vi "GDSIconEditor_MaskIcon.vi"(6 "BgIcon":u8[][](array[numeric]), 8 "ColorsOkayforiconToBeOnTopOf":u8[](array[numeric]), 9 "BgIconOffset":cluster{"X":i32, "Y":i32}, 10 "BgIconMask":u8[](array[numeric]), 11 "IconIn":u8[][](array[numeric])) -> (3 "IconOut":u8[][](array[numeric]))   [LabVIEW 2014]
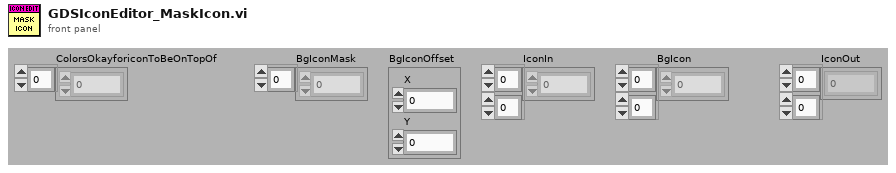
[diagram p1: front panel]
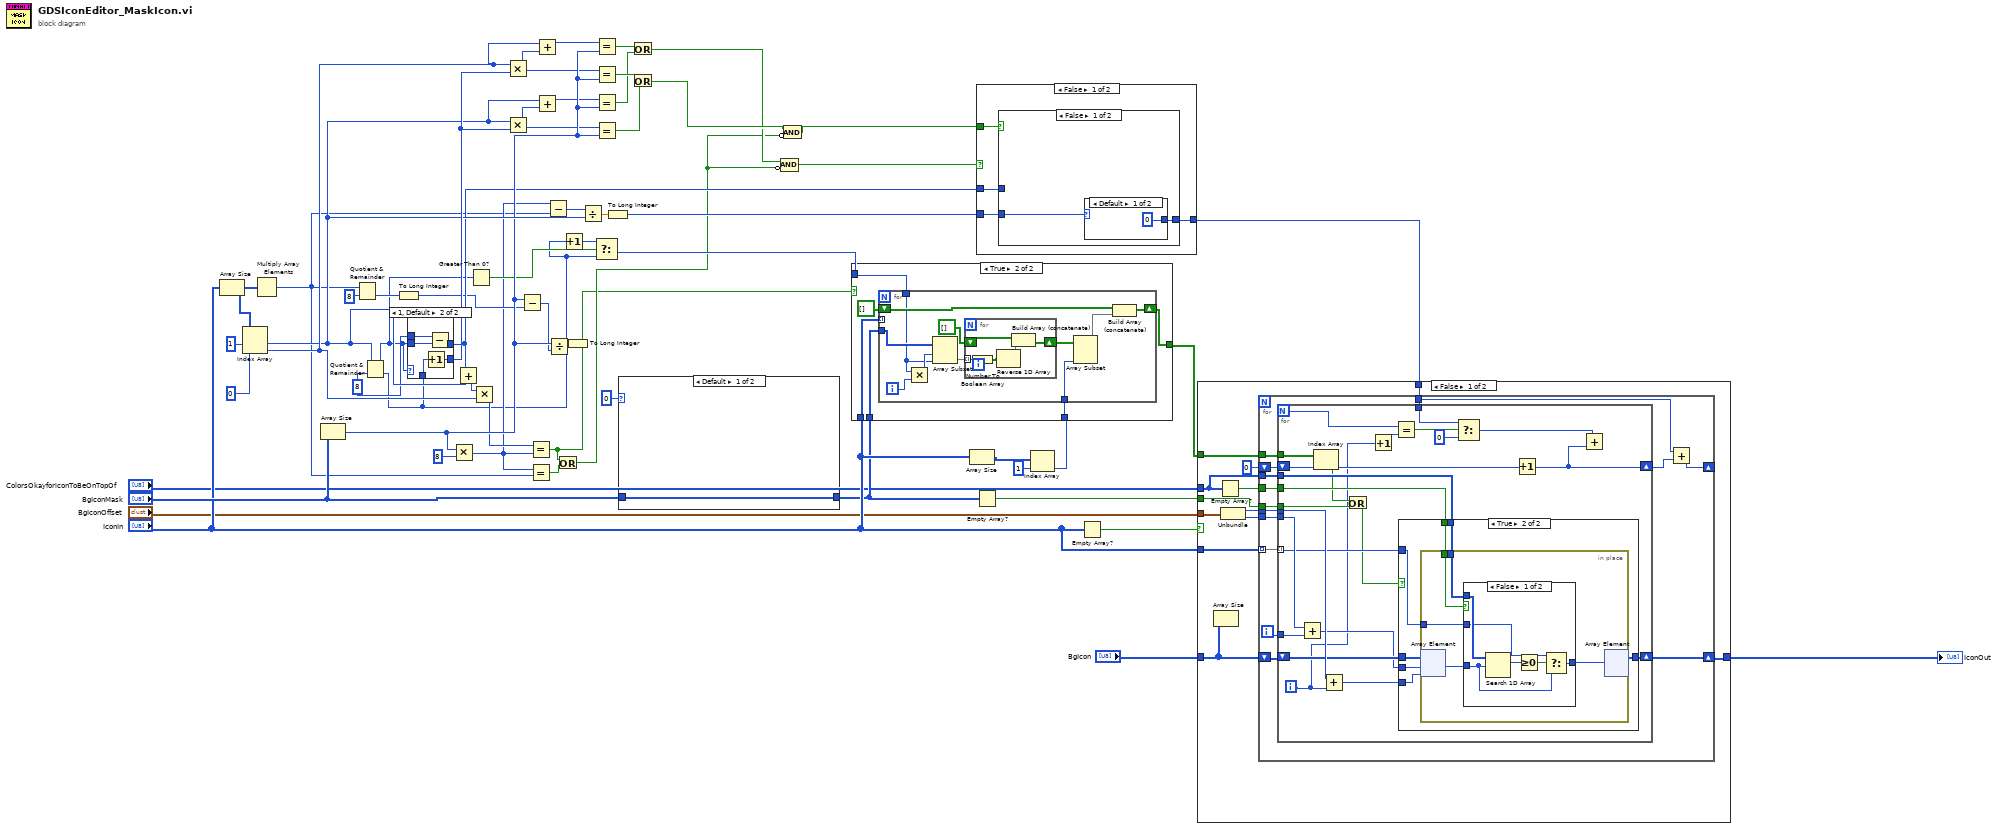
[diagram p0: block diagram]
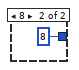
[diagram p2: hidden frame]
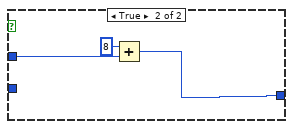
[diagram p4: hidden frame]
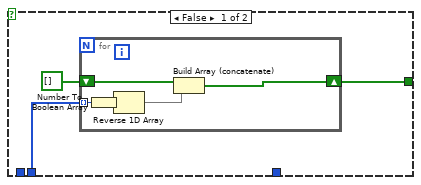
[diagram p6: hidden frame]
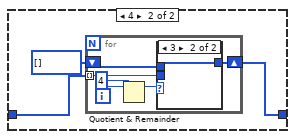
[diagram p7: hidden frame]
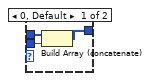
[diagram p8: hidden frame]
diagram:
  w25 = 8 ("y")
  n1 = Array Size(array="IconIn") -> (size(s)=w30:i32[])
  n2 = Index Array(array=w30, index #1=1 ("index"), index #2=0 ("index")) -> (element #1=w48:i32, element #2=w49:i32)
  n3 = Multiply Array Elements(1:w30) -> (0:w6:i32)
  n4 = Array Size(array="BgIconMask") -> (size(s)=w47:i32)
  n5 = Quotient & Remainder(x=w6, y=8) -> (floor(x/y)=w35:i32)  [unwired: 1 out]
  n6 = Quotient & Remainder(x=w48, y=w25) -> (x-y*floor(x/y)=w24:i32, floor(x/y)=w2:i32)
  n7 = To Long Integer(number=w35) -> (32bit integer=w32:i32)
  n8 = case shown="1, Default" w24 {
    tunnel: [_ w63] -> w43
    tunnel: w25 -> [_ w62]
    tunnel: w24 -> [_ w61]
    tunnel: w2 -> [w58 w60]
    tunnel: [w58 w59] -> w50
    frame 0 {
    }
    frame 1, Default {
      n9 = Increment(x=w60) -> (x+1=w59:i32)
      n10 = Subtract(x=w62, y=w61) -> (x-y=w63:i32)
    }
  }
  n11 = Multiply(x=w47, y=8) -> (x*y=w7:i32)
  n12 = Add(x=w43, y=w48) -> (x+y=w27:i32)
  n13 = Greater Than 0?(x=w24) -> (x > 0?=w39:bool)
  n14 = Multiply(x=w27, y=w49) -> (x*y=w26:i32)
  n15 = Multiply(x=w49, y=w50) -> (x*y=w46:i32)
  n16 = Multiply(x=w48, y=w50) -> (x*y=w40:i32)
  n17 = Subtract(x=w47, y=w32) -> (x-y=w34:i32)
  n18 = Equal?(x=w26, y=w7) -> (x = y?=w3:bool)
  n19 = Equal?(x=w7, y=w6) -> (x = y?=w5:bool)
  n20 = Add(x=w49, y=w46) -> (x+y=w45:i32)
  n21 = Add(x=w48, y=w40) -> (x+y=w41:i32)
  n22 = Subtract(x=w7, y=w6) -> (x-y=w18:i32)
  n23 = Divide(x=w47, y=w34) -> (x/y=w33:dbl)
  n24 = Or(x=w3, y=w5) -> (x .or. y?=w4:bool)
  n25 = Increment(x=w2) -> (x+1=w1:i32)
  n26 = To Long Integer(number=w33) -> ()  [unwired: 1 out]
  n27 = Divide(x=w18, y=w48) -> (x/y=w17:dbl)
  n28 = Select(t=w1, s=w39, f=w2) -> (s? t:f=w20:i32)
  n29 = Equal?(x=w45, y=w47) -> (x = y?=w51:bool)
  n30 = Equal?(x=w46, y=w47) -> (x = y?=w54:bool)
  n31 = Equal?(x=w41, y=w47) -> (x = y?=w52:bool)
  n32 = Equal?(x=w40, y=w47) -> (x = y?=w55:bool)
  n33 = To Long Integer(number=w17) -> (32bit integer=w19:i32)
  n34 = case shown="Default" 0 {
    tunnel: "BgIconMask" -> [w64 w67]
    tunnel: [w64 w65] -> w15
    frame Default {
    }
    frame 4 {
      n35 = for {
        tunnel: w67 -> [w73] mode=indexing
        shift-right: [w71] -> w65
        shift-left: u8[] [] -> [w72]
        i -> [w70]
        n36 = Quotient & Remainder(x=w70, y=4) -> (x-y*floor(x/y)=w68:i32)  [unwired: 1 out]
        n37 = case shown="3" w68 {
          tunnel: w73 -> [w76 _]
          tunnel: w72 -> [w75 w77]
          tunnel: [w74 w77] -> w71
          frame 0, Default {
            n38 = Build Array (concatenate)(w75, w76) -> (w74:u8[])
          }
          frame 3 {
          }
        }
      }
    }
  }
  n39 = Or(x=w51, y=w52) -> (x .or. y?=w53:bool)
  n40 = Or(x=w54, y=w55) -> (x .or. y?=w56:bool)
  n41 = Compound Arithmetic op=AND(w53, invert w4) -> (w42:bool)
  n42 = Compound Arithmetic op=AND(w56, invert w4) -> (w44:bool)
  n43 = Array Size(array="IconIn") -> (size(s)=w22:i32[])
  n44 = Empty Array?(array=w15) -> (empty?=w11:bool)
  n45 = case shown="False" w42 {
    tunnel: [w81 w87] -> w16
    tunnel: w19 -> [w80 _]
    tunnel: w43 -> [w78 w89]
    tunnel: w44 -> [w79 _]
    frame False {
      n46 = case shown="False" w79 {
        tunnel: [w83 w86] -> w81
        tunnel: w80 -> [w82 _]
        tunnel: w78 -> [_ w86]
        frame False {
          n47 = case shown="Default" w82 {
            tunnel: [0 8] -> w83
            frame Default {
            }
            frame 8 {
            }
          }
        }
        frame True {
        }
      }
    }
    frame True {
      n48 = Add(x=8, y=w89) -> (x+y=w87:i32)
    }
  }
  n49 = Index Array(array=w22, index=1) -> (element=w23:i32)
  n50 = case shown="True" w3 {
    tunnel: [w92 w101] -> w14
    tunnel: w15 -> [w91 w100]
    tunnel: w20 -> [_ w99]
    tunnel: "IconIn" -> [_ w103]
    tunnel: w23 -> [_ w98]
    frame False {
      n51 = for {
        tunnel: w91 -> [w94] mode=indexing
        shift-right: [w95] -> w92
        shift-left: bool[] [] -> [w97]
        n52 = Number To Boolean Array(number=w94) -> (Boolean array=w96:bool[])
        n53 = Reverse 1D Array(array=w96) -> (reversed array=w93:bool[])
        n54 = Build Array (concatenate)(w97, w93) -> (w95:bool[])
      }
    }
    frame True {
      n55 = for {
        tunnel: w103 -> [_] mode=indexing
        shift-right: [w113] -> w101
        shift-left: bool[] [] -> [w114]
        tunnel: w100 -> [w111]
        tunnel: w99 -> [w109]
        tunnel: w98 -> [w104]
        i -> [w112]
        n56 = Multiply(x=w109, y=w112) -> (x*y=w110:i32)
        n57 = Array Subset(array=w111, index=w110, length=w109) -> (w108:u8[])
        n58 = for {
          tunnel: w108 -> [w118] mode=indexing
          shift-right: [w115] -> w106
          shift-left: bool[] [] -> [w116]
          n59 = Number To Boolean Array(number=w118) -> (Boolean array=w119:bool[])
          n60 = Reverse 1D Array(array=w119) -> (reversed array=w117:bool[])
          n61 = Build Array (concatenate)(w116, w117) -> (w115:bool[])
        }
        n62 = Array Subset(array=w106, length=w104) -> (w105:bool[])  [unwired: 1 in]
        n63 = Build Array (concatenate)(w114, w105) -> (w113:bool[])
      }
    }
  }
  n64 = Empty Array?(array="IconIn") -> (empty?=w9:bool)
  n65 = case shown="False" w9 {
    tunnel: "BgIcon" -> [w131 w189]
    tunnel: [w130 w189] -> w13
    tunnel: "IconIn" -> [w129 _]
    tunnel: "BgIconOffset" -> [w128 _]
    tunnel: "ColorsOkayforiconToBeOnTopOf" -> [w124 _]
    tunnel: w14 -> [w123 _]
    tunnel: w11 -> [w121 _]
    tunnel: w16 -> [w120 _]
    frame False {
      n66 = Array Size(array=w131) -> ()  [unwired: 1 out]
      n67 = Empty Array?(array=w124) -> (empty?=w125:bool)
      n68 = Unbundle(w128) -> ("X"=w126:i32, "Y"=w127:i32)
      n69 = for {
        shift-right: [w144] -> w130
        shift-left: w131 -> [w145]
        tunnel: w129 -> [w143] mode=indexing
        tunnel: w127 -> [w141]
        tunnel: w126 -> [w140]
        tunnel: w125 -> [w139]
        tunnel: w124 -> [w138]
        tunnel: w123 -> [w137]
        shift-right: [w132] -> _
        shift-left: 0 -> [w136]
        tunnel: w121 -> [w135]
        tunnel: w120 -> [w134]
        i -> [w142]
        n70 = for {
          N -> [w150]
          shift-right: [w159] -> w144
          shift-left: w145 -> [w165]
          tunnel: w143 -> [w160] mode=indexing
          tunnel: w142 -> [w168]
          tunnel: w141 -> [w167]
          tunnel: w140 -> [w166]
          tunnel: w139 -> [w162]
          tunnel: w138 -> [w161]
          tunnel: w137 -> [w158]
          shift-right: [w146] -> w133
          shift-left: w136 -> [w157]
          tunnel: w135 -> [w156]
          tunnel: w134 -> [w147]
          i -> [w149]
          n71 = Add(x=w167, y=w168) -> (x+y=w164:i32)
          n72 = Index Array(array=w158, index=w157) -> (element=w155:bool)
          n73 = Add(x=w166, y=w149) -> (x+y=w163:i32)
          n74 = Or(x=w155, y=w156) -> (x .or. y?=w154:bool)
          n75 = Increment(x=w149) -> (x+1=w151:i32)
          n76 = Equal?(x=w150, y=w151) -> (x = y?=w148:bool)
          n77 = case shown="True" w154 {
            tunnel: w165 -> [w169 w176]
            tunnel: w164 -> [_ w175]
            tunnel: w163 -> [_ w174]
            tunnel: w162 -> [_ w173]
            tunnel: w161 -> [_ w172]
            tunnel: w160 -> [_ w171]
            tunnel: [w169 w170] -> w159
            frame False {
            }
            frame True {
              n78 = in-place {
                in-place-border: w173 -> [w181]
                in-place-border: w172 -> [w179]
                in-place-border: w171 -> [w178]
                n79 = in-place-array #1(w176, w175, w174) -> (w180:u8)
                n80 = case shown="False" w181 {
                  tunnel: w180 -> [w183 _]
                  tunnel: w179 -> [w187 _]
                  tunnel: w178 -> [w184 w188]
                  tunnel: [w182 w188] -> w177
                  frame False {
                    n81 = Search 1D Array(1D array=w187, element=w183) -> (index of element=w186:i32)  [unwired: 1 in]
                    n82 = Greater Or Equal To 0?(x=w186) -> (x >= 0?=w185:bool)
                    n83 = Select(t=w184, s=w185, f=w183) -> (s? t:f=w182:u8)
                  }
                  frame True {
                  }
                }
                n84 = in-place-array #1(w177) -> (w170:u8[][])  [unwired: 2 out]
              }
            }
          }
          n85 = Select(t=w147, s=w148, f=0) -> (s? t:f=w152:i32)
          n86 = Increment(x=w157) -> (x+1=w146:i32)
          n87 = Add(x=w152, y=w146) -> ()  [unwired: 1 out]
        }
        n88 = Add(x=w134, y=w133) -> (x+y=w132:i32)
      }
    }
    frame True {
    }
  }
  "IconOut" <- w13
